vi "createdatafile.vi"(8 "error in (no error)":errorcluster, 9 "Save Wheel":bool, 10 "path":path, 11 "QuadraturePositionDecoder in":refnum<class "QuadraturePositionDecoder.lvclass">) -> (0 "error out":errorcluster, 3 "QuadraturePositionDecoder out":refnum<class "QuadraturePositionDecoder.lvclass">)   [LabVIEW 2014, in "QuadraturePositionDecoder.lvclass"]
uses:
  QuadraturePositionDecoder.lvclass
  QuadraturePositionDecoder.lvclass/QuadraturePositionDecoder.ctl
  private/HDF5Tools32/LabView/Create Dataset 2D Double.vi
  private/HDF5Tools32/LabView/HDF5Tools.lvlib
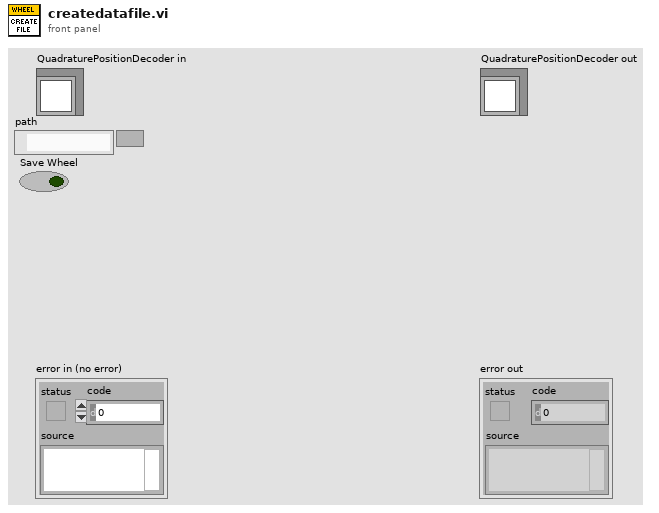
[diagram p1: front panel]
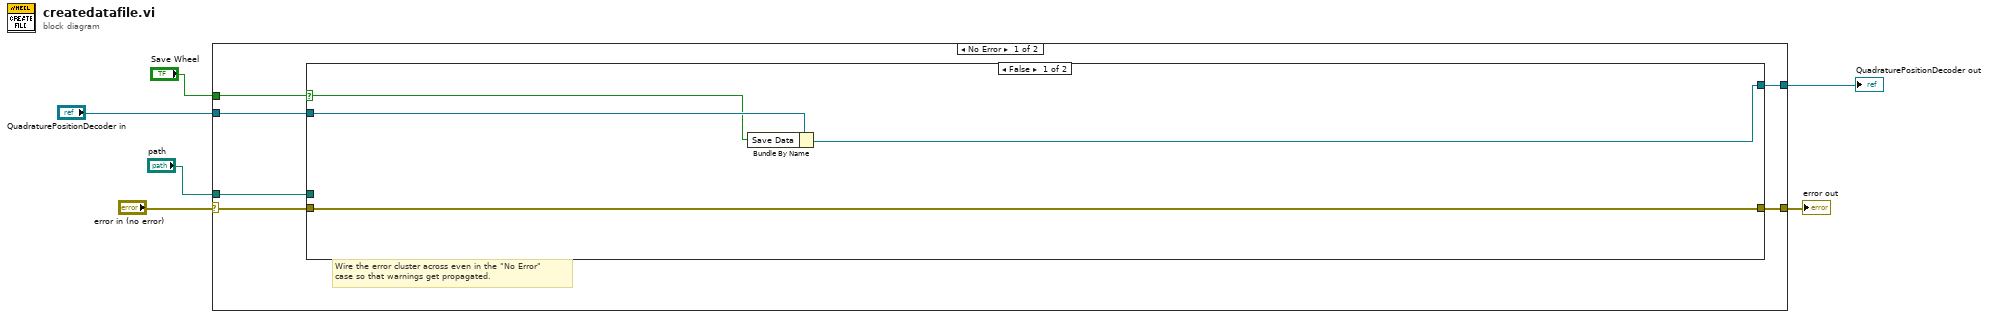
[diagram p0: block diagram]
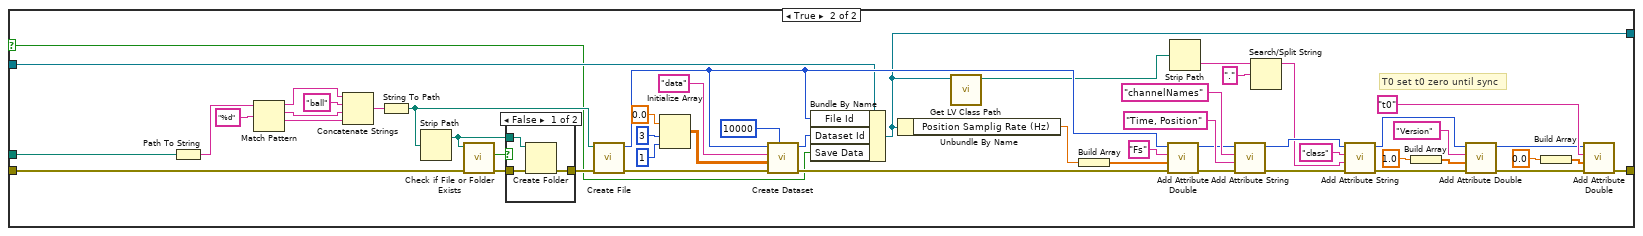
[diagram p2: hidden frame]
diagram:
  n1 = case shown="No Error" "error in (no error)" {
    selector: "error in (no error)" -> [w11 w74]
    tunnel: [w9 w74] -> w5
    tunnel: [w10 w73] -> w3
    tunnel: "QuadraturePositionDecoder in" -> [w12 w73]
    tunnel: "path" -> [w8 _]
    tunnel: "Save Wheel" -> [w7 _]
    frame No Error {
      # "Wire the error cluster across even in the \"No Error\"\ncase so that warnings get propagated."
      n2 = case shown="False" w7 {
        selector: w7 -> [w13 w17]
        tunnel: [w14 w52] -> w10
        tunnel: [w16 w39] -> w9
        tunnel: w12 -> [w15 w19]
        tunnel: w11 -> [w16 w20]
        tunnel: w8 -> [_ w18]
        frame False {
          n3 = Bundle By Name(cluster=w15, "Save Data"=w13) -> (w14:refnum<class "QuadraturePositionDecoder.lvclass">)
        }
        frame True {
          # "T0 set t0 zero until sync"
          n4 = Path To String(path=w18) -> (string=w31:string)
          n5 = Match Pattern(string=w31, regular expression="%d") -> (before substring=w29:string, match substring=w27:string, after substring=w26:string)  [unwired: 1 in, 1 out]
          n6 = Concatenate Strings(w29, "ball" ("string"), w27, w26) -> (w25:string)
          n7 = String To Path(string=w25) -> (path=w24:path)
          n8 = Strip Path(path=w24) -> (stripped path=w23:path)  [unwired: 1 out]
          n9 = call <vilib>:"Check if File or Folder Exists.vi"("error in (no error)"=w20, "path"=w23) -> ("error out"=w21:errorcluster, "file or folder exists?"=w22:bool)  [unwired: 7 in, 1 out]
          n10 = case shown="False" w22 {
            tunnel: w23 -> [w71 _]
            tunnel: w21 -> [w70 w72]
            tunnel: [w69 w72] -> w37
            frame False {
              n11 = Create Folder(path (use dialog)=w71, error in=w70) -> (error out=w69:errorcluster)  [unwired: 1 in, 2 out]
            }
            frame True {
            }
          }
          n12 = call "Create File.vi"("Error in"=w37, "File Name"=w24) -> ("Error out"=w68:errorcluster, "file_id"=w58:i32)  [unwired: 6 in]
          n13 = Initialize Array(0.0, 3 ("dimension size"), 1 ("dimension size")) -> (w63:dbl[][])
          n14 = call-poly "Create Dataset.vi"("Chunk size"=10000, "error in (no error)"=w68, "Datatype"=w63, "Dataset name"="data", "Location id in"=w58) -> ("error out"=w57:errorcluster, "Dataset id"=w62:i32)  [unwired: 5 in]
          n15 = Bundle By Name(cluster=w19, "File Id"=w58, "Dataset Id"=w62, "Save Data"=w17) -> (w52:refnum<class "QuadraturePositionDecoder.lvclass">)
          n16 = Unbundle By Name(w52) -> ("Position Samplig Rate (Hz)"=w35:dbl)
          n17 = call <vilib>:"Get LV Class Path.vi"("object"=w52) -> ("class path"=w55:path)  [unwired: 9 in, 1 out]
          n18 = Build Array(w35) -> (w60:dbl[])
          n19 = call "Add Attribute Double.vi"("error in (no error)"=w57, "data"=w60, "Attribute name"="Fs", "loc_id"=w58) -> ("error out"=w32:errorcluster, "loc_id_out"=w33:i32)  [unwired: 6 in]
          n20 = Strip Path(path=w55) -> (name=w54:string)  [unwired: 1 out]
          n21 = call "Add Attribute String.vi"("error in (no error)"=w32, "Attribute data"="Time, Position", "Attribute name"="channelNames", "loc_id"=w33) -> ("error out"=w50:errorcluster, "loc_id_out"=w56:i32)  [unwired: 6 in]
          n22 = Search/Split String(string=w54, search string/char (-)=".") -> (substring before match=w49:string)  [unwired: 1 in, 2 out]
          n23 = call "Add Attribute String.vi"("error in (no error)"=w50, "Attribute data"=w49, "Attribute name"="class", "loc_id"=w56) -> ("error out"=w46:errorcluster, "loc_id_out"=w44:i32)  [unwired: 6 in]
          n24 = Build Array(1.0) -> (w45:dbl[])
          n25 = call "Add Attribute Double.vi"("error in (no error)"=w46, "data"=w45, "Attribute name"="Version", "loc_id"=w44) -> ("error out"=w41:errorcluster, "loc_id_out"=w40:i32)  [unwired: 6 in]
          n26 = Build Array(0.0 ("element")) -> (w42:dbl[])
          n27 = call "Add Attribute Double.vi"("error in (no error)"=w41, "data"=w42, "Attribute name"="t0", "loc_id"=w40) -> ("error out"=w39:errorcluster)  [unwired: 6 in, 1 out]
        }
      }
    }
    frame Error {
    }
  }
  "error out" <- w5
  "QuadraturePositionDecoder out" <- w3
